vi "Initialize.vi"(7 "Serial Configuration":T1={"Baud Rate"=115200, "Parity"=0, "Data Bits"=8, "Stop Bits"=10, "Flow Control"=0} {"Flow Control" items=["None", "XON/XOFF", "RTS/CTS", "XON/XOFF & RTS/CTS", "DTR/DSR", "XON/XOFF & DTR/DSR"]; "Stop Bits" items=["1.0"=10, "1.5"=15, "2.0"=20]; "Data Bits" items=["7"=7, "8"=8]; "Parity" items=["None", "Odd", "Even", "Mark", "Space"]; "Baud Rate" items=["300"=300, "600"=600, "1200"=1200, "2400"=2400, "4800"=4800, "9600"=9600, "19200"=19200]}, 8 "error in (no error)":errorcluster, 10 "ID Query (True)":bool=TRUE, 11 "VISA resource name":refnum<visa-resource-name>) -> (0 "error out":errorcluster, 3 "VISA resource name out":refnum<visa-resource-name>)   [LabVIEW 2012, in "Roboteq.lvlib"]
doc: "Establishes communication with the sensor and optionally performs a sensor identification query. Therefore, call this VI before calling other sensor driver VIs for this sensor. Generally, you need to call the Initialize VI only once at the beginning of an application."
uses:
  Roboteq.lvlib
panel:
  out "error out 2":errorcluster
  out "read buffer":string
  # "(c) 2010 National Instruments.  ALL RIGHTS RESERVED."
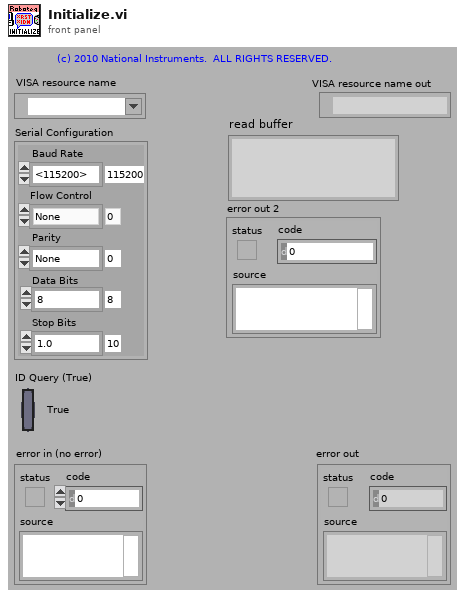
[diagram p1: front panel]
types:
  T1 = cluster{"Baud Rate":u32, "Parity":u16, "Data Bits":u16, "Stop Bits":u16, "Flow Control":u16}
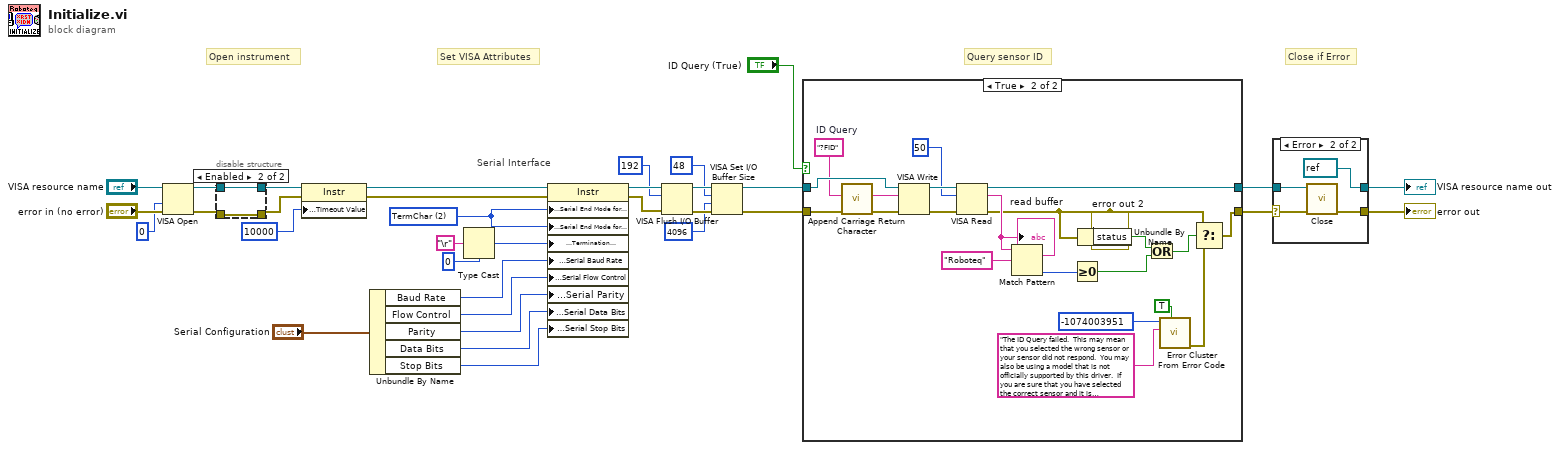
[diagram p0: block diagram]
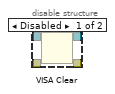
[diagram p2: hidden frame]
diagram:
  w8 = u16 2 items=["None", "LastBit", "TermChar"] ("Serial Settings:Serial End Mode for Reads")
  # "Serial Interface"
  # "Set VISA Attributes"
  # "Close if Error"
  # "Query sensor ID"
  # "Open instrument"
  n1 = VISA Open(access mode=u32 0, error in (no error)="error in (no error)", VISA resource name="VISA resource name") -> (VISA resource name=w25:refnum<visa-resource-name>, error out=w24:errorcluster)  [unwired: 2 in]
  n2 = disable-structure shown="Enabled" {
    disable-tunnel: w25 -> [w38 w40]
    disable-tunnel: w24 -> [w37 w39]
    disable-tunnel: [w36 w40] -> w23
    disable-tunnel: [w35 w39] -> w22
    frame Disabled {
      n3 = VISA Clear(VISA resource name=w38, error in (no error)=w37) -> (VISA resource name out=w36:refnum<visa-resource-name>, error out=w35:errorcluster)
    }
    frame Enabled {
    }
  }
  n4 = property class="Instr"(reference=w23, error in=w22, "General Settings:Timeout Value"=u32 10000) -> (reference out=w28:refnum<visa-resource-name>, error out=w27:errorcluster)
  n5 = Unbundle By Name("Serial Configuration") -> ("Baud Rate"=w6:u32, "Flow Control"=w2:u16, "Parity"=w4:u16, "Data Bits"=w5:u16, "Stop Bits"=w1:u16)
  n6 = Type Cast(type=u8 0, x="\r") -> (*(type *) &x=w7:u8)
  n7 = property class="Instr"(reference=w28, error in=w27, "Serial Settings:Serial End Mode for Reads"=w8, "Serial Settings:Serial End Mode for Writes"=w8, "Message Based Settings:Termination Character"=w7, "Serial Settings:Serial Baud Rate"=w6, "Serial Settings:Serial Flow Control"=w2, "Serial Settings:Serial Parity"=w4, "Serial Settings:Serial Data Bits"=w5, "Serial Settings:Serial Stop Bits"=w1) -> (reference out=w14:refnum<visa-resource-name>, error out=w16:errorcluster)
  n8 = VISA Flush I/O Buffer(VISA resource name=w14, mask (16)=u16 192, error in (no error)=w16) -> (VISA resource name out=w17:refnum<visa-resource-name>, error out=w15:errorcluster)
  n9 = VISA Set I/O Buffer Size(VISA resource name=w17, mask (16)=u16 48, size (4096)=u32 4096 ("size (0)"), error in (no error)=w15) -> (VISA resource name out=w30:refnum<visa-resource-name>, error out=w29:errorcluster)
  n10 = case shown="True" "ID Query (True)" {
    tunnel: [w41 w63] -> w18
    tunnel: [w42 w61] -> w19
    tunnel: w30 -> [w42 w62]
    tunnel: w29 -> [w41 w47]
    frame False {
    }
    frame True {
      w45 = "?FID"  # ID Query
      n11 = call "Append Carriage Return Character.vi"("error in (no error)"=w47, "Command"=w45) -> ("error out"=w46:errorcluster, "Command Out"=w43:string)  [unwired: 8 in]
      n12 = VISA Write(VISA resource name=w62, write buffer=w43, error in (no error)=w46) -> (VISA resource name out=w59:refnum<visa-resource-name>, error out=w44:errorcluster)  [unwired: 1 out]
      n13 = VISA Read(VISA resource name=w59, byte count=u32 50, error in (no error)=w44) -> (VISA resource name out=w61:refnum<visa-resource-name>, read buffer=w60:string, error out=w51:errorcluster)  [unwired: 1 out]
      "read buffer" <- w60
      "error out 2" <- w51
      n14 = Match Pattern(string=w60, regular expression="Roboteq") -> (offset past match=w52:i32)  [unwired: 1 in, 3 out]
      n15 = Greater Or Equal To 0?(x=w52) -> (x >= 0?=w49:bool)
      n16 = Unbundle By Name(w51) -> ("status"=w50:bool)
      n17 = Or(x=w50, y=w49) -> (x .or. y?=w48:bool)
      n18 = call <vilib>:"Error Cluster From Error Code.vi"("show call chain? (False)"=TRUE, "error message (\"\")"="The ID Query failed.  This may mean that you selected the wrong sensor or your sensor did not respond.  You may also be using a model that is not officially supported by this driver.  If you are sure that you have selected the correct sensor and it is responding, try disabling the ID Query." ("Source (VI Name)"), "error code (0)"=-1074003951 ("Code")) -> ("error out"=w56:errorcluster)  [unwired: 6 in]
      n19 = Select(t=w51, s=w48, f=w56) -> (s? t:f=w63:errorcluster)
    }
  }
  n20 = case shown="Error" w18 {
    selector: w18 -> [w64 w67]
    tunnel: w19 -> [w65 w68]
    tunnel: [w65 refnum<visa-resource-name> refnum ("VISA resource name out")] -> w21
    tunnel: [w64 w69] -> w20
    frame No Error {
    }
    frame Error {
      n21 = call "Close.vi"("error in (no error)"=w67, "VISA resource name"=w68) -> ("error out"=w69:errorcluster)  [unwired: 9 in]
    }
  }
  "VISA resource name out" <- w21
  "error out" <- w20
